vi "例4-13.vi"() -> ()   [LabVIEW 2019]
panel:
  in  "列长度":dbl=2.0
  in  "列索引":dbl=1.0
  in  "行长度":dbl=2.0
  in  "行索引":dbl=1.0
  out "输出数组":dbl[][](array[numeric]) format="%_4g"
  in  "输入数组":dbl[][](array[numeric]) format="%4_4g"
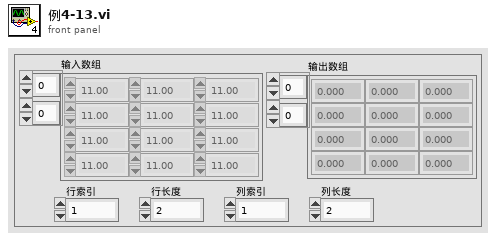
[diagram p1: front panel]
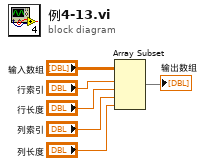
[diagram p0: block diagram]
diagram:
  n1 = Array Subset(array="输入数组", index (row)="行索引", length (row)="行长度", index (col)="列索引", length (col)="列长度") -> (→"输出数组":dbl[][])
